vi "Set Mmeber Info.vi"(6 "Week(0)":i32, 8 "error in (no error)":errorcluster, 9 "Department(\"\")":string, 10 "Name(\"\")":string, 11 "AttendRecord in":refnum<class "AttendRecord.lvclass">) -> (0 "error out":errorcluster, 3 "AttendRecord out":refnum<class "AttendRecord.lvclass">)   [LabVIEW 2015, in "Admin_Actor.lvlib" / "AttendRecord.lvclass"]
uses:
  AttendRecord.lvclass
  AttendRecord.lvclass/AttendRecord.ctl
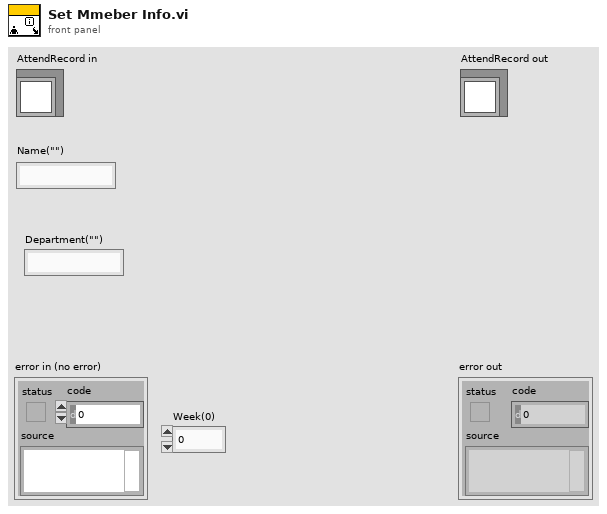
[diagram p1: front panel]
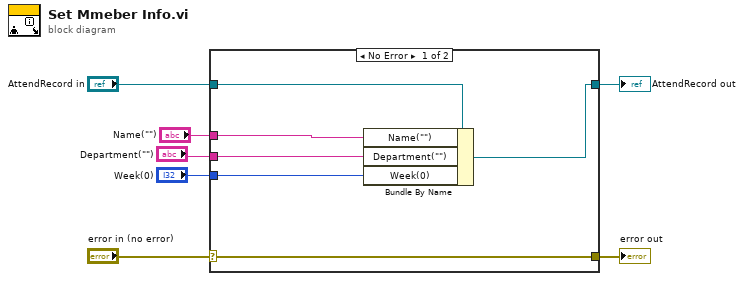
[diagram p0: block diagram]
diagram:
  n1 = case shown="No Error" "error in (no error)" {
    selector: "error in (no error)" -> [w13 w14]
    tunnel: [w13 w14] -> w6
    tunnel: [w11 w15] -> w4
    tunnel: "AttendRecord in" -> [w12 w15]
    tunnel: "Name(\"\")" -> [w10 _]
    tunnel: "Department(\"\")" -> [w9 _]
    tunnel: "Week(0)" -> [w8 _]
    frame No Error {
      n2 = Bundle By Name(cluster=w12, "Name(\"\")"=w10, "Department(\"\")"=w9, "Week(0)"=w8) -> (w11:refnum<class "AttendRecord.lvclass">)
    }
    frame Error {
    }
  }
  "error out" <- w6
  "AttendRecord out" <- w4
